vi "Read Characters From File (no popup).vi"(0 "file path (dialog if empty)":path, 2 "number of characters (all:-1)":i32=-1, 3 "start of read offset (chars.:0)":i32, 5 "convert eol? (no:F)":bool) -> (6 "new file path (NotAPath if cancelled)":path, 7 "character string":string, 8 "EOF?":bool, 9 "mark after read (chars.)":i32)   [LabVIEW 2011]
doc: "LabVIEW no longer supports this VI. Use the Read Text function instead. Reads a specified number of characters from a byte stream file beginning at a specified character offset. The VI opens the file before reading from it and closes it afterwards."
panel:
  out "error out":errorcluster
  in  "prompt":string="Choose file to read."
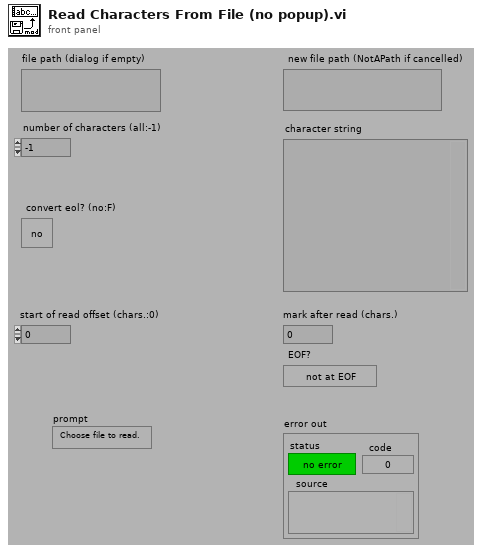
[diagram p1: front panel]
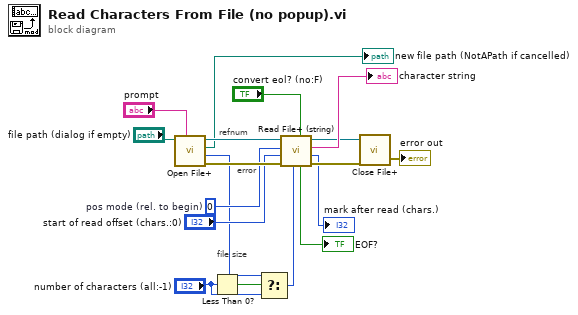
[diagram p0: block diagram]
diagram:
  w15 = i16 0  # pos mode (rel. to begin)
  # "file size"
  # "error"
  # "refnum"
  n1 = call <vilib>:"Open File+.vi"("prompt"="prompt", "file path (\" \")"="file path (dialog if empty)") -> ("error out"=w17:errorcluster, "file size (bytes)"=w6:i32, "file path"=→"new file path (NotAPath if cancelled)":path, "refnum"=w9:refnum<file>)  [unwired: 6 in]
  n2 = Less Than 0?(x="number of characters (all:-1)") -> (x < 0?=w7:bool)
  n3 = Select(t=w6, s=w7, f="number of characters (all:-1)") -> (s? t:f=w4:i32)
  n4 = call <vilib>:"Read File+ (string).vi"("convert eol? (no:F)"="convert eol? (no:F)", "count"=w4, "error in (no error)"=w17, "pos offset (bytes:0)"="start of read offset (chars.:0)", "pos mode (rel. to current:2)"=w15, "refnum"=w9) -> ("error out"=w13:errorcluster, "mark after read (bytes)"=→"mark after read (chars.)":i32, "string"=→"character string":string, "dup refnum"=w12:refnum<file>, "EOF?"=→"EOF?":bool)  [unwired: 1 in]
  n5 = call <vilib>:"Close File+.vi"("error in (no error)"=w13, "refnum"=w12) -> ("error out"=→"error out":errorcluster)  [unwired: 3 in, 2 out]
